vi "Initialise Accelerometer.vi"(8 "error in (no error)":errorcluster, 11 "LSM9DS1 IMU in":refnum<class "LSM9DS1 IMU.lvclass">) -> (0 "error out":errorcluster, 3 "LSM9DS1 IMU out":refnum<class "LSM9DS1 IMU.lvclass">)   [LabVIEW 2020, in "LSM9DS1 IMU.lvclass"]
uses:
  LSM9DS1 IMU.lvclass
  LSM9DS1 IMU.lvclass/LSM9DS1 IMU.ctl
  Read Accel & Gyro I2C.vi
  Write Accel & Gyro I2C.vi
  LINX I2C/LINX I2C.lvclass
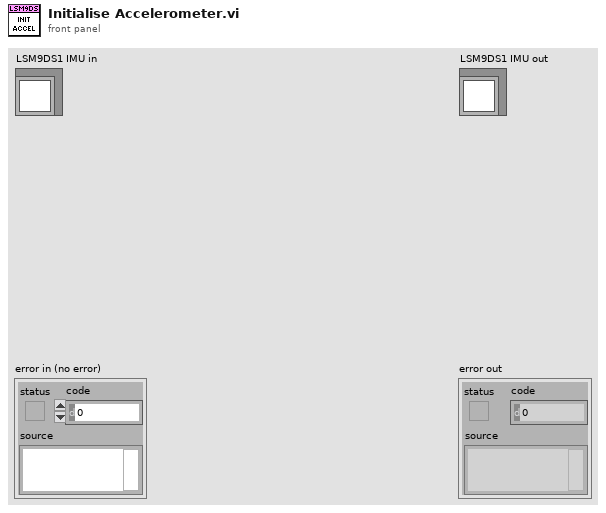
[diagram p1: front panel]
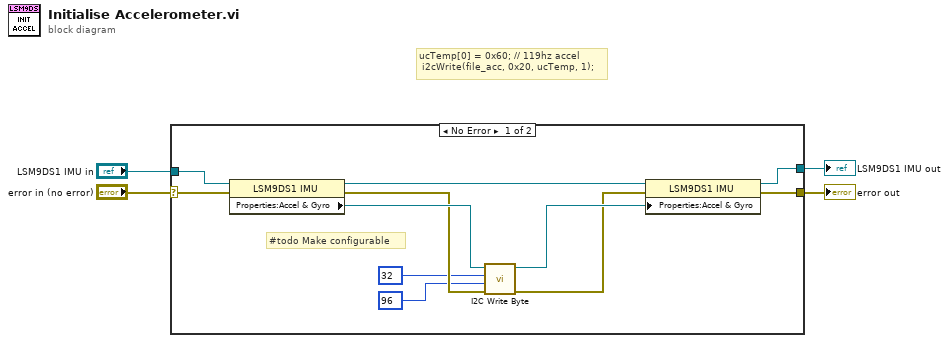
[diagram p0: block diagram]
diagram:
  # "ucTemp[0] = 0x60; // 119hz accel\n\ti2cWrite(file_acc, 0x20, ucTemp, 1);"
  n1 = case shown="No Error" "error in (no error)" {
    selector: "error in (no error)" -> [w10 w17]
    tunnel: [w9 w17] -> w3
    tunnel: [w12 w16] -> w1
    tunnel: "LSM9DS1 IMU in" -> [w15 w16]
    frame No Error {
      # "#todo Make configurable"
      n2 = property class="LSM9DS1 IMU"(reference=w15, error in=w10) -> (reference out=w13:refnum<class "LSM9DS1 IMU.lvclass">, error out=w11:errorcluster, "Properties:Accel & Gyro"=w14:refnum<class "LINX I2C.lvclass">)
      n3 = call "I2C Write Byte.vi"("error in (no error)"=w11, "Value"=u8 96 ("I2C Slave Address 2"), "Register Address"=u8 32 ("I2C Slave Address 2"), "LINX I2C in"=w14) -> ("error out"=w5:errorcluster, "LINX I2C out"=w8:refnum<class "LINX I2C.lvclass">)  [unwired: 6 in]
      n4 = property class="LSM9DS1 IMU"(reference=w13, error in=w5, "Properties:Accel & Gyro"=w8) -> (reference out=w12:refnum<class "LSM9DS1 IMU.lvclass">, error out=w9:errorcluster)
    }
    frame Error {
    }
  }
  "error out" <- w3
  "LSM9DS1 IMU out" <- w1
